vi "Retreive Ball.vi"(9 "SolenoidDevRef":T1={"DevStatus"={"status"=FALSE, "code"=0, "source"=""}, "Pneumatics Control Module"=0, "Forward Solenoid Channel"=enum."Invalid", "Reverse Solenoid Channel"=enum."Invalid"}, 11 "Iteration":i32) -> (1 "Speed":dbl, 3 "Finished":bool)   [LabVIEW 2016]
uses:
  <vilib>/Rock Robotics/WPI/Solenoid/WPI_SolenoidDevRef.ctl
  <vilib>/Rock Robotics/WPI/Solenoid/WPI_SolenoidChannel.ctl
  <vilib>/Rock Robotics/WPI/Solenoid/WPI_SolenoidValue.ctl
  <vilib>/Rock Robotics/WPI/Solenoid/WPI_SolenoidSetEnum.vi
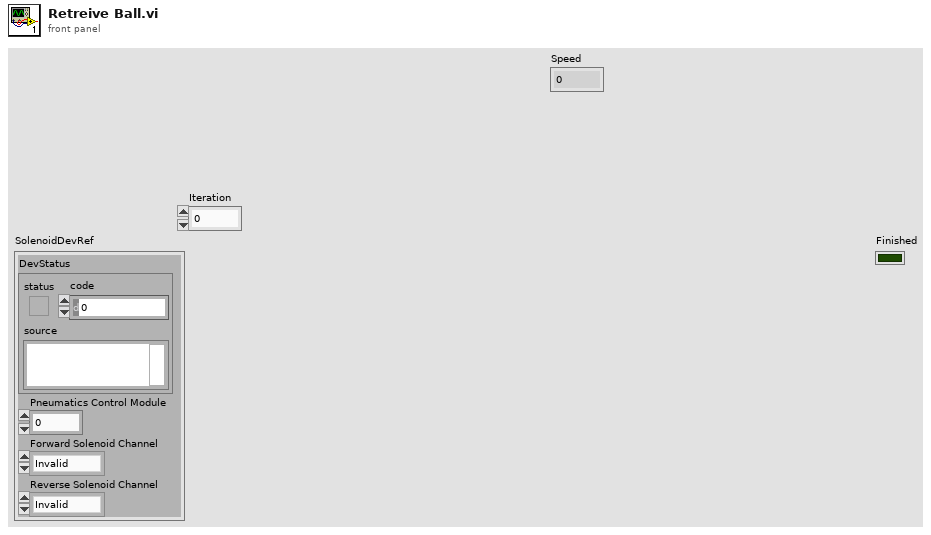
[diagram p1: front panel]
types:
  T1 = typedef "WPI_SolenoidDevRef.ctl" = cluster{"DevStatus":errorcluster, "Pneumatics Control Module":u8, "Forward Solenoid Channel":T2, "Reverse Solenoid Channel":T2}
  T2 = typedef "WPI_SolenoidChannel.ctl" = enum8{"Solenoid 0", "Solenoid 1", "Solenoid 2", "Solenoid 3", "Solenoid 4", "Solenoid 5", "Solenoid 6", "Solenoid 7", "Invalid"}
  T3 = typedef "WPI_SolenoidValue.ctl" = enum16{"Off", "On", "Forward", "Reverse"}
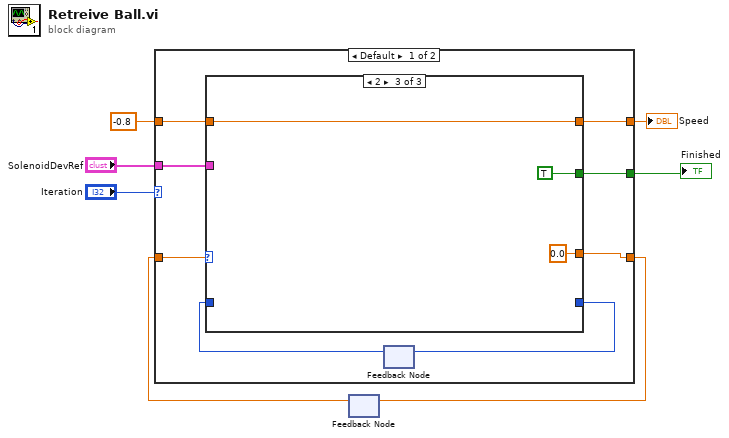
[diagram p0: block diagram]
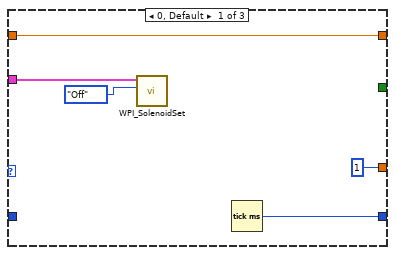
[diagram p2: hidden frame]
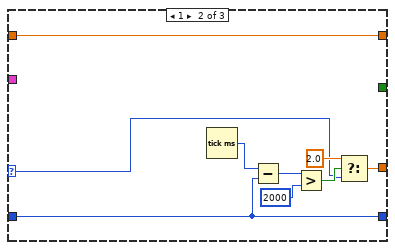
[diagram p3: hidden frame]
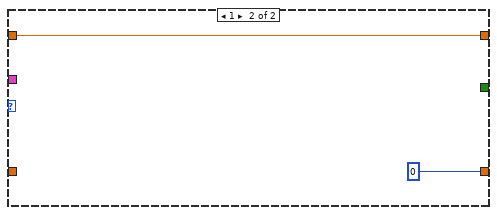
[diagram p4: hidden frame]
diagram:
  n1 = feedback #1() -> (w5:dbl)  [unwired: 1 in]
  n2 = case shown="Default" "Iteration" {
    tunnel: [w10 0] -> w6
    tunnel: w5 -> [w15 _]
    tunnel: -0.8 -> [w14 w33]
    tunnel: [w13 w33] -> w3
    tunnel: "SolenoidDevRef" -> [w9 _]
    tunnel: [w8 _] -> w1
    frame Default {
      n3 = feedback #2() -> (w11:u32)  [unwired: 1 in]
      n4 = case shown="2" w15 {
        selector: w15 -> [_ w22 _]
        tunnel: w14 -> [w18 w21 w31]
        tunnel: [w18 w21 w31] -> w13
        tunnel: [w20 w28 _] -> w12
        tunnel: w11 -> [_ w28 _]
        tunnel: [1 w25 0.0 ("t")] -> w10
        tunnel: w9 -> [w16 _ _]
        tunnel: [_ _ TRUE] -> w8
        frame 0, Default {
          n5 = call-poly <vilib>:"WPI_SolenoidSet.vi"("Value"=WPI_SolenoidValue."Off", "SolenoidDevRef"=w16) -> ()  [unwired: 8 in, 2 out]
          n6 = Tick Count (ms)() -> (millisecond timer value=w20:u32)
        }
        frame 1 {
          n7 = Tick Count (ms)() -> (millisecond timer value=w29:u32)
          n8 = Subtract(x=w29, y=w28) -> (x-y=w27:u32)
          n9 = Greater?(x=w27, y=u32 2000) -> (0:w23:bool)
          n10 = Select(t=2.0, s=w23, f=w22) -> (s? t:f=w25:dbl)
        }
        frame 2 {
        }
      }
      n11 = feedback-in #2(w12) -> ()
    }
    frame 1 {
    }
  }
  "Speed" <- w3
  "Finished" <- w1
  n12 = feedback-in #1(w6) -> ()
